vi "check table array.vi"(8 "OldVal":string[][](array[string]), 11 "NewVal":string[][](array[string])) -> (0 "new tag":bool, 1 "needs dialog":bool, 2 "Column":i32, 3 "Row":i32)   [LabVIEW 2013, in "PL Framework Configuration Tool.lvlib" / "EngineTags.lvclass"]
uses:
  EngineTags.lvclass
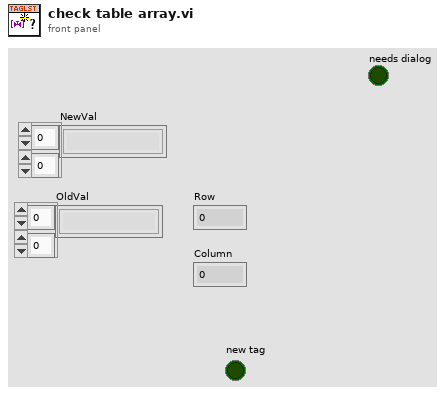
[diagram p1: front panel]
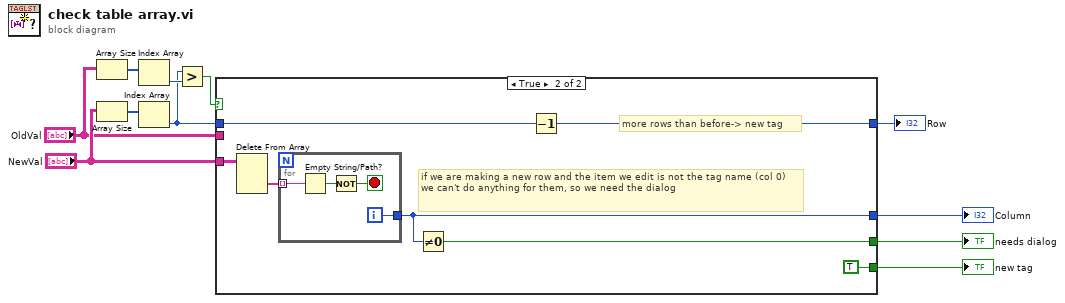
[diagram p0: block diagram]
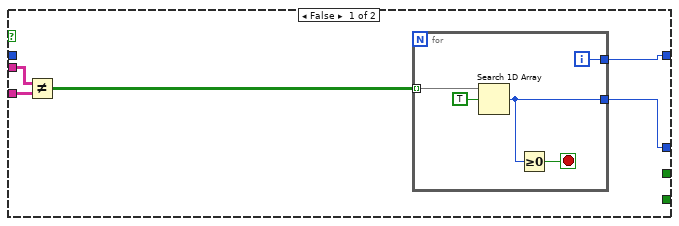
[diagram p2: hidden frame]
diagram:
  n1 = Array Size(array="OldVal") -> (size(s)=w7:i32[])
  n2 = Array Size(array="NewVal") -> (size(s)=w8:i32[])
  n3 = Index Array(array=w7) -> (element=w5:i32)  [unwired: 1 in]
  n4 = Index Array(array=w8) -> (element=w2:i32)  [unwired: 1 in]
  n5 = Greater?(x=w2, y=w5) -> (0:w4:bool)
  n6 = case shown="True" w4 {
    tunnel: [w15 w22] -> w11
    tunnel: [w14 w24] -> w10
    tunnel: "NewVal" -> [w13 w27]
    tunnel: "OldVal" -> [w12 _]
    tunnel: [_ TRUE] -> w3
    tunnel: w2 -> [_ w25]
    tunnel: [_ w23] -> w1
    frame False {
      n7 = Not Equal?(x=w12, y=w13) -> (x != y?=w16:bool[][])
      n8 = for {
        tunnel: w16 -> [w21] mode=indexing
        tunnel: [w19] -> w15
        tunnel: [w18] -> w14
        i -> [w19]
        stop <- w17 stop-if-true
        n9 = Search 1D Array(1D array=w21, element=TRUE) -> (index of element=w18:i32)  [unwired: 1 in]
        n10 = Greater Or Equal To 0?(x=w18) -> (x >= 0?=w17:bool)
      }
    }
    frame True {
      # "if we are making a new row and the item we edit is not the tag name (col 0) we can't do anything for them, so we need the dialog"
      # "more rows than before-> new tag"
      n11 = Delete From Array(array=w27) -> (deleted portion=w26:string[])  [unwired: 3 in, 1 out]
      n12 = for {
        tunnel: w26 -> [w32] mode=indexing
        tunnel: [w30] -> w24
        i -> [w30]
        stop <- w29 stop-if-true
        n13 = Empty String/Path?(string/path=w32) -> (empty?=w31:bool)
        n14 = Not(x=w31) -> (.not. x?=w29:bool)
      }
      n15 = Not Equal To 0?(x=w24) -> (x != 0?=w23:bool)
      n16 = Decrement(x=w25) -> (x-1=w22:i32)
    }
  }
  "Column" <- w10
  "Row" <- w11
  "new tag" <- w3
  "needs dialog" <- w1
